vi "runTestScenario.vi"(0 "Constant Analog Output Voltage Test  in":refnum<class "Constant Current Output Test.lvclass">, 5 "ILC":refnum<class "ILC.lvclass">, 11 "error in (no error)":errorcluster) -> (4 "Constant Analog Output Voltage Test  out":refnum<class "Constant Current Output Test.lvclass">, 6 "ILC 2":refnum<class "ILC.lvclass">, 8 "TestExecution":T2, 10 "Result":T1, 15 "error out":errorcluster)   [LabVIEW 2015, in "Constant Current Output Test.lvclass"]
uses:
  Constant Current Output Test.lvclass
  Typedefs/TestExecution.ctl
  Typedefs/PassFailTest.ctl
  <userlib>/Common/ILC/ILC/ILC.lvclass
  Typedefs/WriteLogMessageInput.ctl
  Typedefs/TestScenarioTypes.ctl
  Typedefs/WriteDataFileInput.ctl
  Constant Current Output Test.lvclass/Constant Current Output Test.ctl
  Model/TestLog/ITestLog/ITestLog.lvclass
  Typedefs/ILCBTTypedefs.lvlib
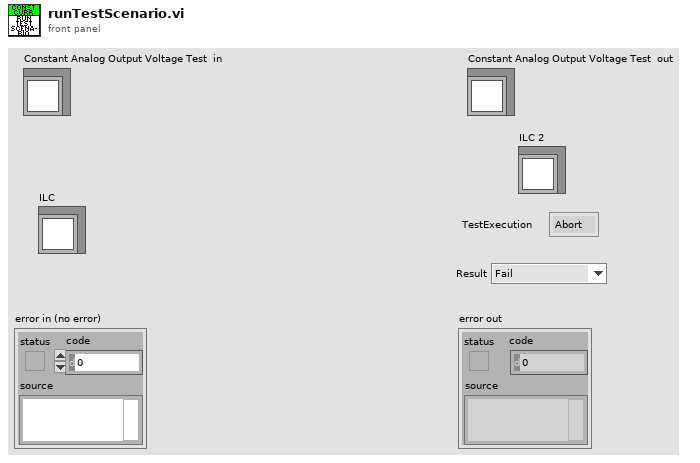
[diagram p1: front panel]
types:
  T1 = typedef "ILCBTTypedefs.lvlib/PassFailTest.ctl" = enum16{"Fail", "Pass", "NA"}
  T2 = typedef "ILCBTTypedefs.lvlib/TestExecution.ctl" = enum16{"Abort", "Continue"}
  T3 = typedef "ILCBTTypedefs.lvlib/WriteDataFileInput.ctl" = cluster{"Test Scenario":T4, "File Name":string, "Output":string[]}
  T4 = typedef "ILCBTTypedefs.lvlib/TestScenarioTypes.ctl" = enum16{"+3.3VD", "+5.1V", "+24V", "RELVALV1", "RELVALV2", "Verify DAC_A = -1.00A", "Verify DAC_A = -0.75A", "Verify DAC_A = -0.50A", "Verify DAC_A = -0.25A", "Verify DAC_A = 0.00A", "Verify DAC_A = 0.25A", "Verify DAC_A = 0.50A", "Verify DAC_A = 0.75A", "Verify DAC_A = 1.00A", "Verify DAC_B = -1.00A", "Verify DAC_B = -0.75A", "Verify DAC_B = -0.50A", "Verify DAC_B = -0.25A", "Verify DAC_B = 0.00A", "Verify DAC_B = 0.25A", "Verify DAC_B = 0.50A", "Verify DAC_B = 0.75A", "Verify DAC_B = 1.00A"}
  T5 = typedef "ILCBTTypedefs.lvlib/WriteLogMessageInput.ctl" = cluster{"Test Scenario":T4, "Description":string, "Actual Value":string, "Data File":string, "Result":T1}
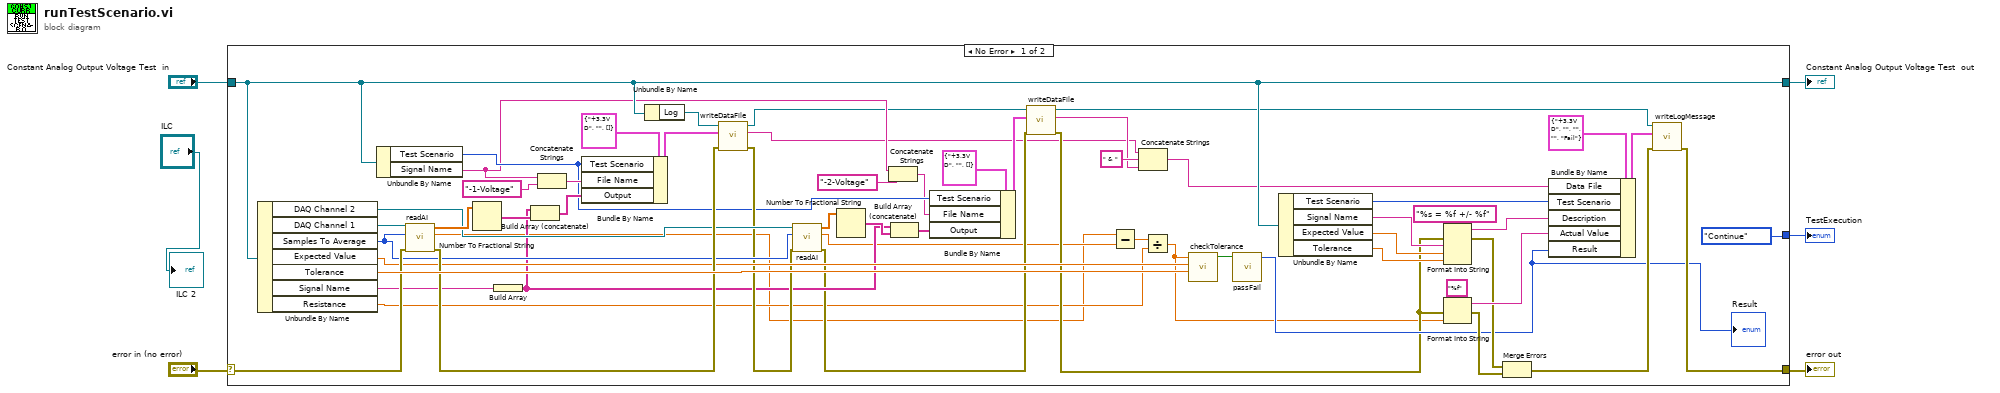
[diagram p0: block diagram]
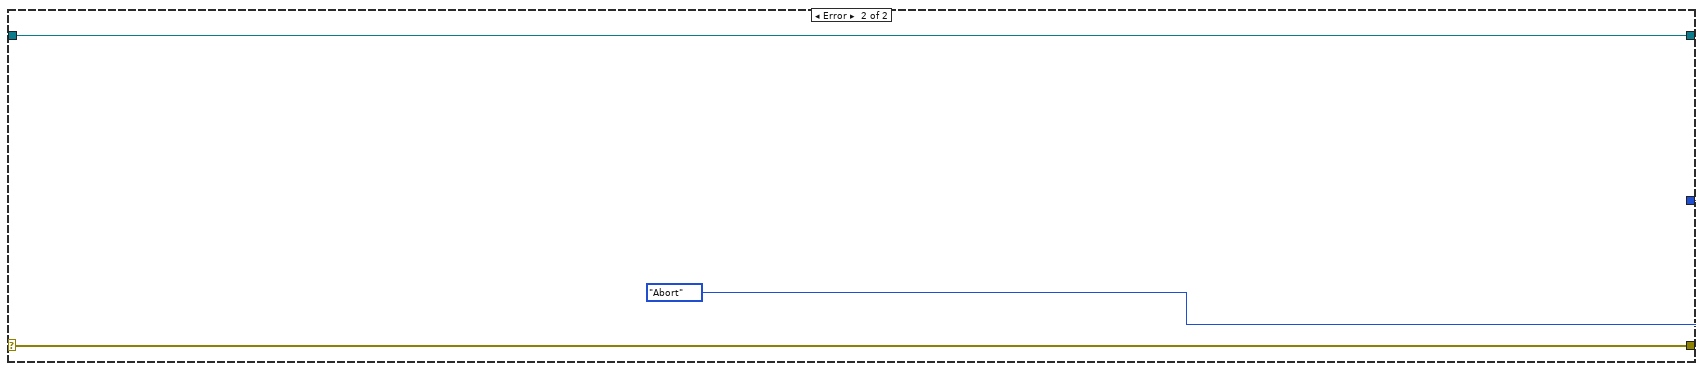
[diagram p2: hidden frame]
diagram:
  n1 = case shown="No Error" "error in (no error)" {
    selector: "error in (no error)" -> [w47 w67]
    tunnel: [w42 w67] -> w5
    tunnel: [TestExecution."Continue" ("TestExecution") TestExecution."Abort" ("TestExecution")] -> w4
    tunnel: "Constant Analog Output Voltage Test  in" -> [w41 w65]
    tunnel: [w41 w65] -> w2
    frame No Error {
      n2 = Unbundle By Name(w41) -> ("DAQ Channel 2"=w33:refnum<k21>, "DAQ Channel 1"=w64:refnum<k21>, "Samples To Average"=w32:i32, "Expected Value"=w34:dbl, "Tolerance"=w59:dbl, "Signal Name"=w35:string, "Resistance"=w11:dbl)
      n3 = Unbundle By Name(w41) -> ("Test Scenario"=w26:T4, "Signal Name"=w24:string)
      n4 = call "readAI.vi"("error in (no error)"=w47, "Samples To Read"=w32, "DAQ Channel To Read"=w64) -> ("error out"=w46:errorcluster, "Average"=w9:dbl, "Samples"=w40:dbl[])  [unwired: 6 in]
      n5 = Number To Fractional String(number=w40) -> (F-format string=w37:string[])  [unwired: 3 in]
      n6 = Build Array(w35) -> (w28:string[])
      n7 = Build Array (concatenate)(w28, w37) -> (w36:string[])
      n8 = Concatenate Strings(w24, "-1-Voltage" ("string")) -> (w60:string)
      n9 = Bundle By Name(cluster=T3 {"Test Scenario"=enum."+3.3VD", "File Name"="", "Output"=[]} ("WriteDataFileInput"), "Test Scenario"=w26, "File Name"=w60, "Output"=w36) -> (w61:T3)
      n10 = Unbundle By Name(w41) -> ("Log"=w63:refnum<class "ITestLog.lvclass">)
      n11 = call-dynamic "writeDataFile.vi"("error in (no error)"=w46, "WriteDataFileInput"=w61, "ITestLog in"=w63) -> ("error out"=w31:errorcluster, "Relative Path"=w14:string, "ITestLog out"=w20:refnum<class "ITestLog.lvclass">)  [unwired: 6 in]
      n12 = call "readAI.vi"("error in (no error)"=w31, "Samples To Read"=w32, "DAQ Channel To Read"=w33) -> ("error out"=w18:errorcluster, "Average"=w10:dbl, "Samples"=w30:dbl[])  [unwired: 6 in]
      n13 = Number To Fractional String(number=w30) -> (F-format string=w29:string[])  [unwired: 3 in]
      n14 = Concatenate Strings(w24, "-2-Voltage" ("string")) -> (w23:string)
      n15 = Build Array (concatenate)(w28, w29) -> (w27:string[])
      n16 = Bundle By Name(cluster=T3 {"Test Scenario"=enum."+3.3VD", "File Name"="", "Output"=[]} ("WriteDataFileInput"), "Test Scenario"=w26, "File Name"=w23, "Output"=w27) -> (w21:T3)
      n17 = call-dynamic "writeDataFile.vi"("error in (no error)"=w18, "WriteDataFileInput"=w21, "ITestLog in"=w20) -> ("error out"=w17:errorcluster, "Relative Path"=w15:string, "ITestLog out"=w19:refnum<class "ITestLog.lvclass">)  [unwired: 6 in]
      n18 = Subtract(x=w9, y=w10) -> (x-y=w12:dbl)
      n19 = Concatenate Strings(w14, " & " ("string"), w15) -> (w13:string)
      n20 = Divide(x=w12, y=w11) -> (x/y=w8:dbl)
      n21 = call "checkTolerance.vi"("Tolerance"=w59, "Expected Value"=w34, "Average"=w8) -> ("Boolean"=w56:bool)  [unwired: 8 in]
      n22 = call "passFail.vi"("Boolean"=w56) -> ("Result"=w39:T1)  [unwired: 10 in]
      "Result" <- w39
      n23 = Unbundle By Name(w41) -> ("Test Scenario"=w55:T4, "Signal Name"=w53:string, "Expected Value"=w52:dbl, "Tolerance"=w51:dbl)
      n24 = Format Into String(format string="%s = %f +/- %f", error in=w17, w53, w52, w51) -> (resulting string=w50:string, error out=w45:errorcluster)  [unwired: 1 in]
      n25 = Format Into String(format string="%f", error in=w17, w8) -> (resulting string=w48:string, error out=w44:errorcluster)  [unwired: 1 in]
      n26 = Merge Errors(w45, w44) -> (w43:errorcluster)
      n27 = Bundle By Name(cluster=T5 {"Test Scenario"=enum."+3.3VD", "Description"="", "Actual Value"="", "Data File"="", "Result"=enum."Fail"} ("WriteLogMessageInput"), "Data File"=w13, "Test Scenario"=w55, "Description"=w50, "Actual Value"=w48, "Result"=w39) -> (w57:T5)
      n28 = call-dynamic "writeLogMessage.vi"("error in (no error)"=w43, "WriteLogMessageInput"=w57, "ITestLog in"=w19) -> ("error out"=w42:errorcluster)  [unwired: 7 in, 1 out]
    }
    frame Error {
    }
  }
  "Constant Analog Output Voltage Test  out" <- w2
  "error out" <- w5
  "TestExecution" <- w4
  "ILC 2" <- "ILC"
